vi "Get Minimum Log Level.vi"(11 "Logger in":refnum<class "Logger.lvclass">) -> (2 "minimum log level":T1, 3 "Logger out":refnum<class "Logger.lvclass">)   [LabVIEW 2018, in "GLog.lvlib" / "Logger.lvclass"]
uses:
  Logger.lvclass
  Log Levels.ctl
  Logger.lvclass/Logger.ctl
  GLog.lvlib
panel:
  # "Connector Pane"
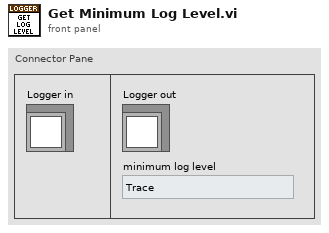
[diagram p1: front panel]
types:
  T1 = typedef "GLog.lvlib/Log Levels.ctl" = enum16{"Trace", "Debug", "Info", "Warning", "Error", "Critical"}
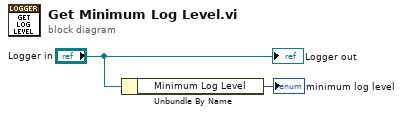
[diagram p0: block diagram]
diagram:
  n1 = Unbundle By Name("Logger in") -> ("Minimum Log Level"=→"minimum log level":T1)
  "Logger out" <- "Logger in"
